vi "Get Enqueuer ID from Actor.vi"(11 "Actor":refnum<class "Actor.lvclass">) -> (2 "Valid Enqueuer?":bool, 3 "Enqueuer ID string out":string)   [LabVIEW 2020]
doc: "Get the unique ID from 'Message Enqueuer'."
uses:
  PPL/HDH.Actor Framework.Core.Actor.lvlibp/1abvi3w/vi.lib/ActorFramework/Actor/Actor.lvclass
  Utility/Utility.lvlib
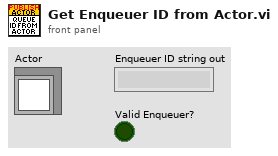
[diagram p1: front panel]
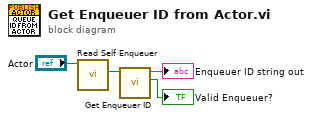
[diagram p0: block diagram]
diagram:
  n1 = call "Read Self Enqueuer.vi"("Actor"="Actor") -> ("Self Enqueuer"=w3:refnum<class "Message Enqueuer.lvclass">)  [unwired: 10 in]
  n2 = call "Get Enqueuer ID.vi"("Message Enqueuer in"=w3) -> ("Valid Enqueuer?"=→"Valid Enqueuer?":bool, "Enqueuer ID string out"=→"Enqueuer ID string out":string)  [unwired: 9 in]
